vi "Abort test.vi"(8 "error in":errorcluster, 11 "Megger cluster in":T1={"Read data"={"Firmware version"="", "Model number"="", "Serial number"=0, "Ramp rate"=0.0, "Test Voltage"=0.0, "Test duration"=0.0, "Test stop watch"=0.0, "measured Current (nA)"=0.0, "calculated Resistance"=0.0, "Test Mode"=enum."Insulation resistance (IR)", "Test status"=enum."Waiting to start test"}, "Connected?"=FALSE, "Device status array"=[]}) -> (0 "error out":errorcluster, 3 "Megger cluster out":T1={"Read data"={"Firmware version"="", "Model number"="", "Serial number"=0, "Ramp rate"=0.0, "Test Voltage"=0.0, "Test duration"=0.0, "Test stop watch"=0.0, "measured Current (nA)"=0.0, "calculated Resistance"=0.0, "Test Mode"=enum."Insulation resistance (IR)", "Test status"=enum."Waiting to start test"}, "Connected?"=FALSE, "Device status array"=[]})   [LabVIEW 2014]
doc: "This function is used to abort a running test."
uses:
  Private/Controls/Megger cluster.ctl
  Private/Controls/Global Megger.vi
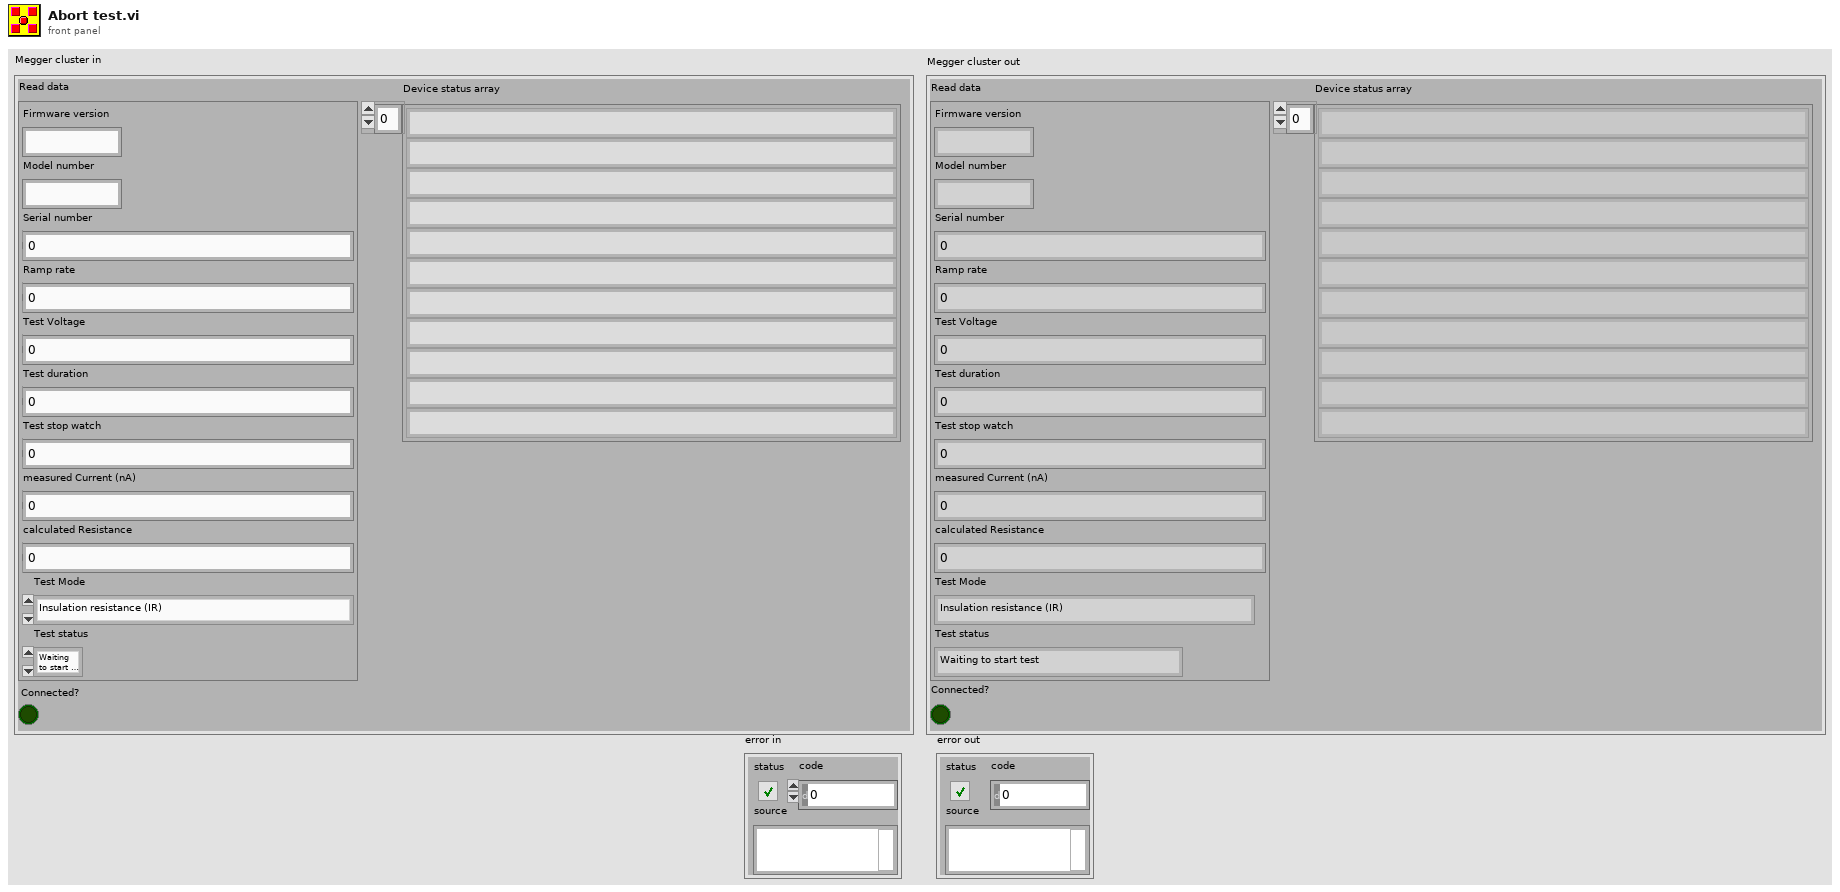
[diagram p1: front panel]
types:
  T1 = typedef "Megger cluster.ctl" = cluster{"Read data":cluster{"Firmware version":string, "Model number":string, "Serial number":i32, "Ramp rate":dbl, "Test Voltage":dbl, "Test duration":sgl, "Test stop watch":sgl, "measured Current (nA)":dbl, "calculated Resistance":dbl, "Test Mode":enum16{"N/A", "Insulation resistance (IR)", "Timed Insulation resistance (IR(t))", "Diaelectric Absorption Ratio (DAR)", "Polarisation Index (PI)", "Diaelectric Dishcharge (DD)", "Step voltage (SV)", "Ramp test (Ramp)"}, "Test status":enum16{"Waiting to start test", "Unable to start test", "Test progressing normally", "Performing post test measurements", "Test has ended normally", "Test has been aborted"}}, "Connected?":bool, "Device status array":string[]}
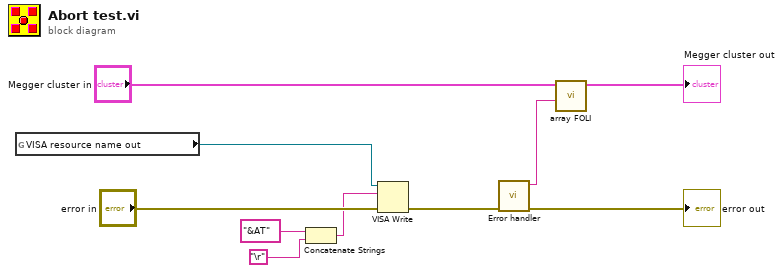
[diagram p0: block diagram]
diagram:
  n1 = global read "Global Megger.vi" "VISA resource name out"() -> (w5:refnum<visa-resource-name>)
  n2 = Concatenate Strings("&AT", "\r") -> (w1:string)
  n3 = VISA Write(VISA resource name=w5, write buffer=w1, error in (no error)="error in") -> (error out=w7:errorcluster)  [unwired: 2 out]
  n4 = call "Error handler.vi"("error in"=w7) -> ("error out"=→"error out":errorcluster, "Status string"=w8:string)  [unwired: 8 in, 1 out]
  n5 = call "array FOLI.vi"("status string"=w8, "Megger cluster in"="Megger cluster in") -> ("Megger cluster out"=→"Megger cluster out":T1)  [unwired: 9 in]
